vi "Demo.vi"() -> ()   [LabVIEW 2018, in "Multicolumn ListBox.lvclass"]
uses:
  Multicolumn ListBox.lvclass
  <vilib>/NI/AMC/Read Termination Message.vi
  <vilib>/NI/AMC/Create Single Message.vi
  <vilib>/NI/AMC/Update Message Routing Info.vi
  <vilib>/NI/AMC/Send Message.vi
  <vilib>/NI/AMC/Globals.vi
  <vilib>/NI/AMC/AMC.lvlib
panel:
  in  "Index":i16=-1
  in  "Rows":string[][](array[string])
  in  "Multicolumn ListBox in":refnum<class "Multicolumn ListBox.lvclass">
  out "status":string
  in  "process":bool
  in  "exit":bool
  in  "Multicolumn Listbox":i32(listbox)
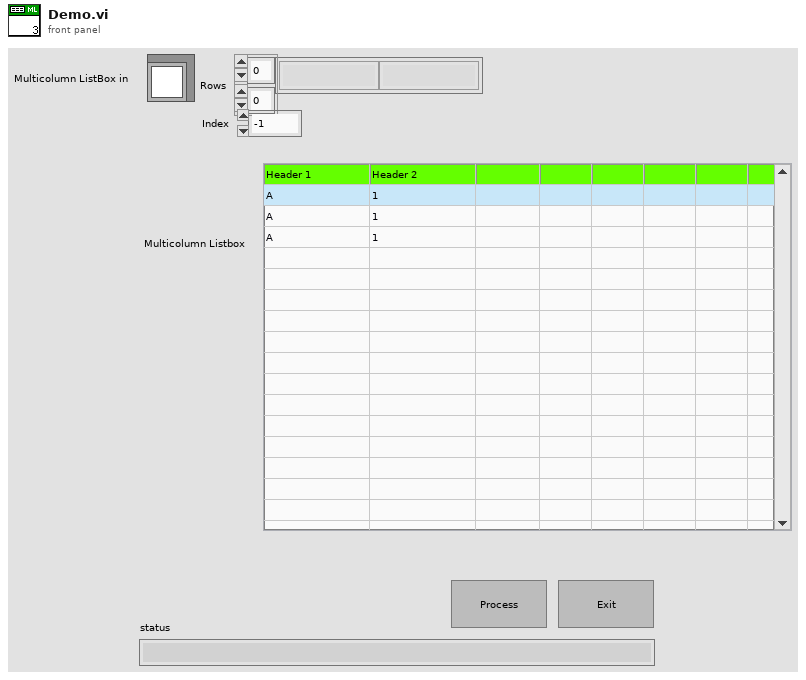
[diagram p1: front panel]
types:
  T1 = cluster{"CurrentFile":path, "status":string, "Multicolumn ListBox out":refnum<class "Multicolumn ListBox.lvclass">}
  T2 = typedef "AMC.lvlib/Message Queue.ctl" = refnum<queue>
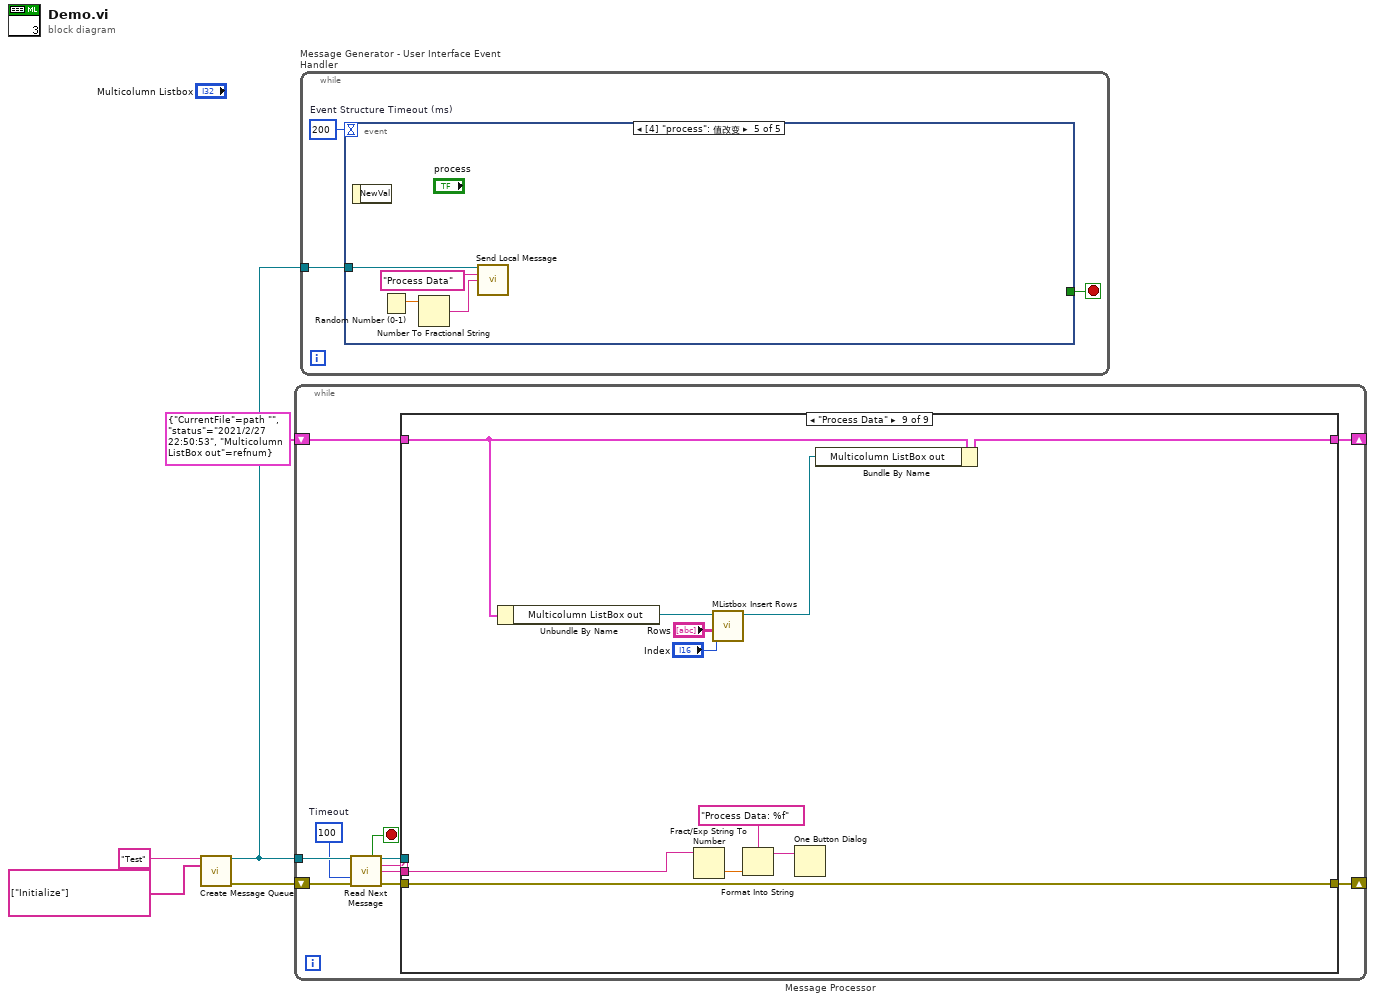
[diagram p0: block diagram]
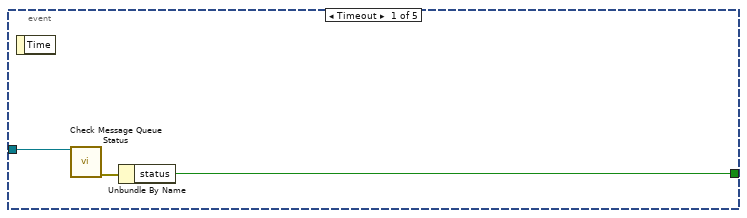
[diagram p2: hidden frame]
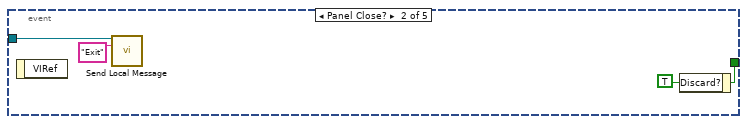
[diagram p3: hidden frame]
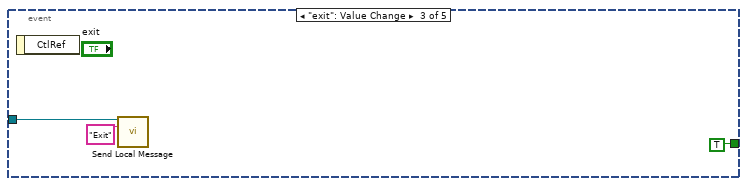
[diagram p4: hidden frame]
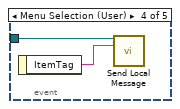
[diagram p5: hidden frame]
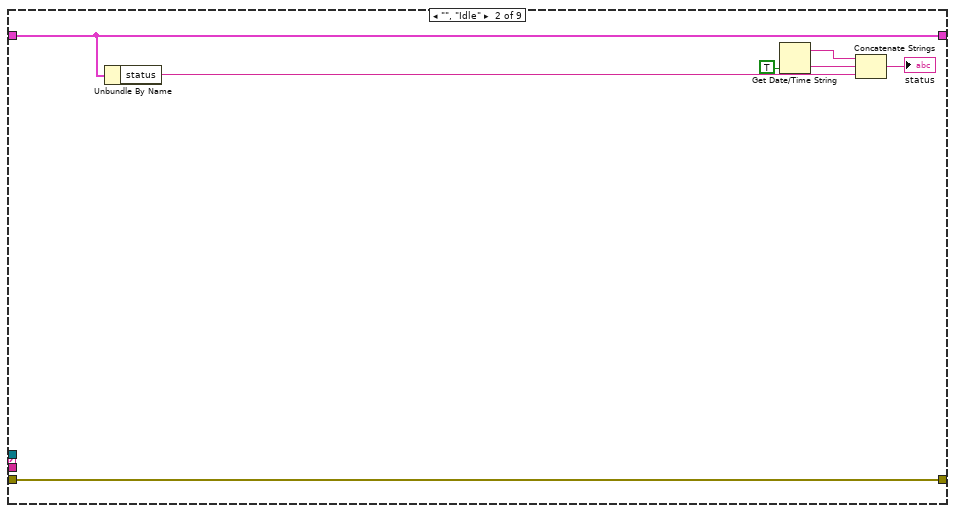
[diagram p7: hidden frame]
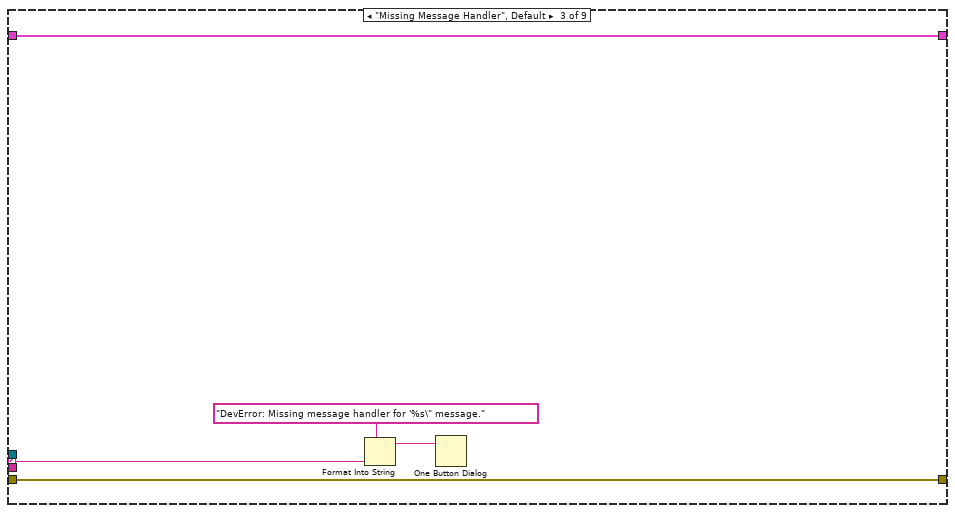
[diagram p8: hidden frame]
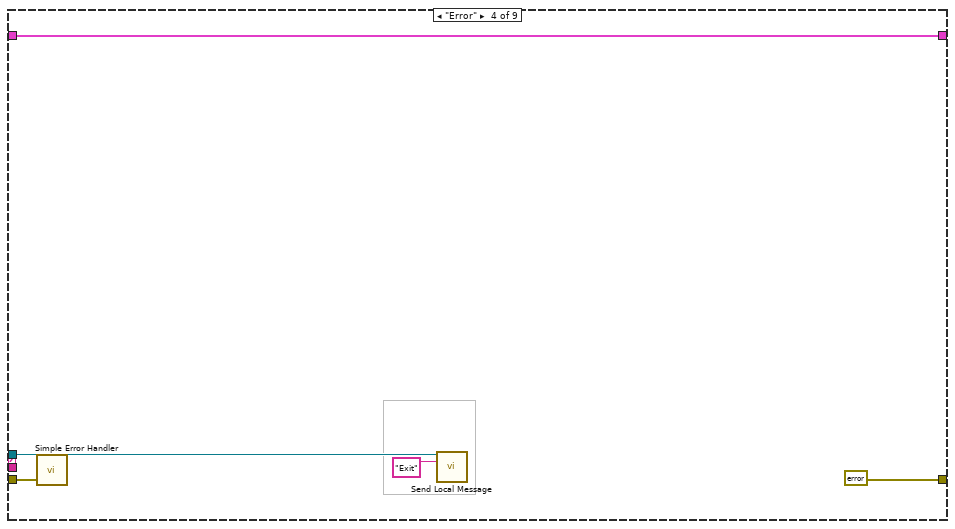
[diagram p9: hidden frame]
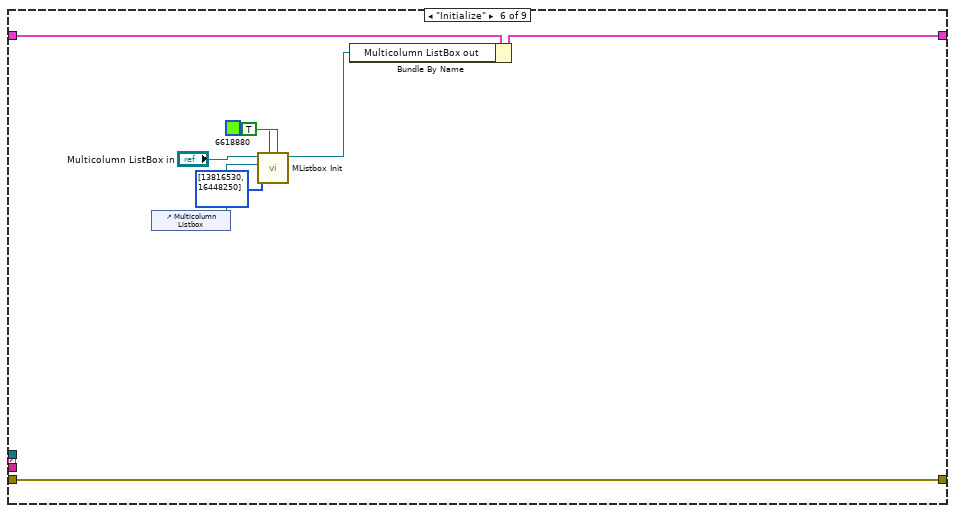
[diagram p11: hidden frame]
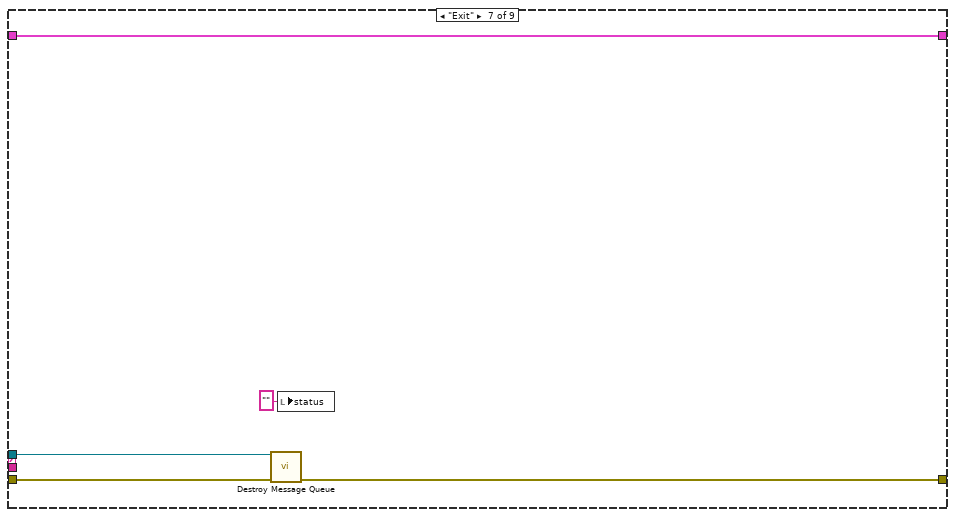
[diagram p12: hidden frame]
diagram:
  n1 = call <vilib>:"Create Message Queue.vi"("message queue name"="Test", "initial message names"=string[] ["Initialize"]) -> ("message queue out"=w3:T2, "error out"=w2:errorcluster)  [unwired: 12 in]
  n2 = while "Message Processor" {
    shift-left: w2 -> [w10]
    shift-right: [w14] -> _
    tunnel: w3 -> [w11]
    shift-left: T1 {"CurrentFile"=path "", "status"="2021/2/27 22:50:53", "Multicolumn ListBox out"=refnum} ("state variables") -> [w16]
    shift-right: [w15] -> _
    stop <- w13 stop-if-true
    w6 = 100  # Timeout
    n3 = call <vilib>:"Read Next Message.vi"("message queue in"=w11, "timeout (1 ms)"=w6, "error in"=w10) -> ("exit process?"=w13:bool, "message queue out"=w12:T2, "message name"=w8:string, "message value"=w7:string, "error out"=w9:errorcluster)  [unwired: 5 in, 3 out]
    n4 = case shown="\"Process Data\"" w8 {
      selector: w8 -> [_ _ w28 _ _ _ _ _ _]
      tunnel: [w18 w21 w30 w35 w37 w43 w51 w53 w55] -> w15
      tunnel: w16 -> [w18 w21 w30 w35 w37 w46 w51 w53 w59]
      tunnel: w12 -> [_ _ _ w33 _ _ w48 _ _]
      tunnel: w9 -> [w17 w25 w29 w31 w36 w45 w49 w52 w64]
      tunnel: [w17 w25 w29 errorcluster {"status"=FALSE, "code"=0, "source"=""} ("error out") w36 w45 w47 w52 w64] -> w14
      tunnel: w7 -> [_ _ _ _ _ _ _ _ w63]
      frame "---------- Framework Operations ----------" {
      }
      frame "", "Idle" {
        n5 = Unbundle By Name(w21) -> ("status"=w19:string)
        n6 = Get Date/Time String(want seconds? (F)=TRUE) -> (date string=w24:string, time string=w20:string)  [unwired: 2 out]
        n7 = Concatenate Strings(w24, w20, w19) -> (→"status":string)
      }
      frame "Missing Message Handler", Default {
        n8 = Format Into String(format string="DevError: Missing message handler for '%s\" message." ("message"), w28) -> (resulting string=w26:string)  [unwired: 2 in, 1 out]
        n9 = One Button Dialog(message=w26) -> ()  [unwired: 2 out]
      }
      frame "Error" {
        n10 = call <vilib>:"Simple Error Handler.vi"("error in (no error)"=w31) -> ()  [unwired: 1 in, 8 out]
        n11 = call <vilib>:"Send Local Message.vi"("message queue in"=w33, "message name"="Exit") -> ()  [unwired: 11 in, 3 out]
      }
      frame "---------- Generic Operations ----------" {
      }
      frame "Initialize" {
        n12 = control-ref of="Multicolumn Listbox"() -> (w44:refnum<vi>)
        n13 = call "MListbox Init.vi"("Select Entire Rows"=TRUE, "Header Backcolor"=u32 6618880, "Row Backcolor"=u32[] [13816530, 16448250], "MListbox Ref"=w44, "Multicolumn ListBox in"="Multicolumn ListBox in") -> ("Multicolumn ListBox out"=w42:refnum<class "Multicolumn ListBox.lvclass">)  [unwired: 5 in, 1 out]
        n14 = Bundle By Name(cluster=w46, "Multicolumn ListBox out"=w42) -> (w43:T1)
      }
      frame "Exit" {
        n15 = call <vilib>:"Destroy Message Queue.vi"("message queue in"=w48, "error in"=w49) -> ("error out"=w47:errorcluster)  [unwired: 11 in, 2 out]
        n16 = local write "status"("" ("Status")) -> ()
      }
      frame "---------- Application Operations ----------" {
      }
      frame "Process Data" {
        n17 = Unbundle By Name(w59) -> ("Multicolumn ListBox out"=w58:refnum<class "Multicolumn ListBox.lvclass">)
        n18 = Fract/Exp String To Number(string=w63) -> (number=w62:dbl)  [unwired: 4 out]
        n19 = call "MListbox Insert Rows.vi"("Rows"="Rows", "Index"="Index", "Multicolumn ListBox in"=w58) -> ("Multicolumn ListBox out"=w54:refnum<class "Multicolumn ListBox.lvclass">)  [unwired: 7 in, 1 out]
        n20 = Format Into String(format string="Process Data: %f" ("message"), w62) -> (resulting string=w60:string)  [unwired: 2 in, 1 out]
        n21 = One Button Dialog(message=w60) -> ()  [unwired: 2 out]
        n22 = Bundle By Name(cluster=w59, "Multicolumn ListBox out"=w54) -> (w55:T1)
      }
    }
  }
  n23 = while "Message Generator - User Interface Event Handler" {
    tunnel: w3 -> [w65]
    stop <- w66 stop-if-true
    w67 = 200  # Event Structure Timeout (ms)
    n24 = event shown="[4] \"process\": 值改变" {
      selector: _ -> [_ _ _ _ _]
      dyn-events: _ -> [_ _ _ _ _]
      timeout: w67 -> [_ _ _ _ _]
      tunnel: [w68 w73 TRUE ("Discard?") _ _] -> w66
      tunnel: w65 -> [w69 w71 w74 w77 w82]
      event Timeout {
        n25 = event-data() -> ()  [unwired: 2 out]
        n26 = call <vilib>:"Check Message Queue Status.vi"("message queue in"=w69) -> ("error out"=w70:errorcluster)  [unwired: 10 in, 4 out]
        n27 = Unbundle By Name(w70) -> ("status"=w68:bool)
      }
      event Panel Close? {
        w73 = TRUE ("Discard?")
        n28 = event-data() -> ()  [unwired: 2 out]
        n29 = call <vilib>:"Send Local Message.vi"("message queue in"=w71, "message name"="Exit") -> ()  [unwired: 11 in, 3 out]
        n30 = event-data("Discard?"=w73) -> ()  [unwired: 1 in, 1 out]
      }
      event "exit": Value Change {
        n31 = event-data() -> ()  [unwired: 2 out]
        n32 = call <vilib>:"Send Local Message.vi"("message queue in"=w74, "message name"="Exit") -> ()  [unwired: 11 in, 3 out]
      }
      event Menu Selection (User) {
        n33 = event-data() -> ("ItemTag"=w78:string)  [unwired: 1 out]
        n34 = call <vilib>:"Send Local Message.vi"("message queue in"=w77, "message name"=w78) -> ()  [unwired: 11 in, 3 out]
      }
      event "process": Value Change {
        n35 = event-data() -> ()  [unwired: 2 out]
        n36 = Random Number (0-1)() -> (number: 0 to 1=w79:dbl)
        n37 = Number To Fractional String(number=w79) -> (F-format string=w80:string)  [unwired: 3 out]
        n38 = call <vilib>:"Send Local Message.vi"("message queue in"=w82, "message name"="Process Data", "message value"=w80) -> ()  [unwired: 10 in, 3 out]
      }
    }
  }
